vi "WinCI IsConnected to Provider.vi"(8 "error in (no error)":errorcluster) -> (0 "error out":errorcluster, 2 "active connection?":bool)   [LabVIEW 2020, in "NI_SCC_WinCI.lvlib"]
uses:
  <vilib>/SourceControl/Providers/WinCI/NI_SCC_WinCI.lvlib
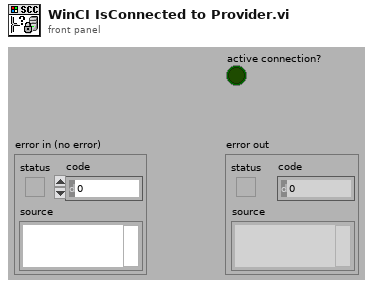
[diagram p1: front panel]
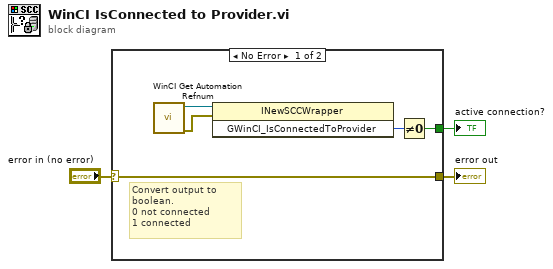
[diagram p0: block diagram]
diagram:
  n1 = case shown="No Error" "error in (no error)" {
    selector: "error in (no error)" -> [w8 w9]
    tunnel: [w8 w9] -> w2
    tunnel: [w7 _] -> w1
    frame No Error {
      # "Convert output to boolean.\n0 not connected\n1 connected"
      n2 = call <vilib>:"WinCI Get Automation Refnum.vi"() -> ("error out"=w4:errorcluster, "automation refnum"=w5:refnum<k7>)  [unwired: 10 out]
      n3 = invoke class="INewSCCWrapper" method="GWinCI_IsConnectedToProvider"(reference=w5, error in=w4) -> ("GWinCI_IsConnectedToProvider"=w6:i32)  [unwired: 1 in, 2 out]
      n4 = Not Equal To 0?(x=w6) -> (x != 0?=w7:bool)
    }
    frame Error {
    }
  }
  "error out" <- w2
  "active connection?" <- w1
